vi "SortColumnEntriesIntoSections.vi"(1 "Array":refnum<class "ClickableText.lvclass">[](array[class])) -> (0 "Sorted Array":T1(array[cluster]))   [LabVIEW 2009, in "NavScreen.lvlib"]
uses:
  NavScreen.lvlib
  Classes/ClickableText/ClickableText.lvclass
  Classes/Link/Link.lvclass
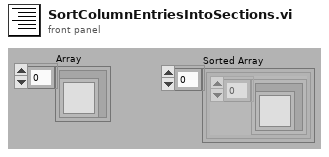
[diagram p1: front panel]
types:
  T1 = cluster{refnum<class "ClickableText.lvclass">[]}[]
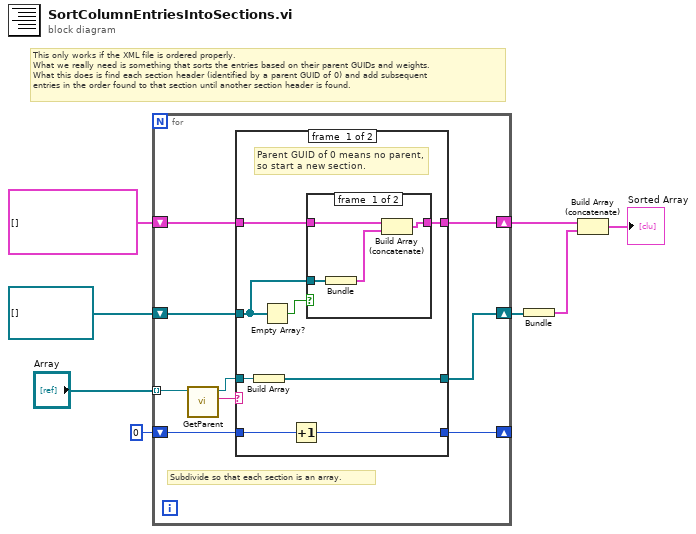
[diagram p0: block diagram]
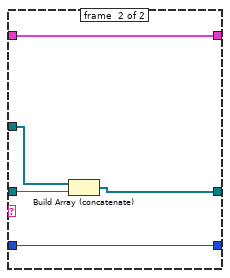
[diagram p3: hidden frame]
diagram:
  # "This only works if the XML file is ordered properly.\nWhat we really need is something that sorts the entries based on their parent GUIDs and weights.\nWhat this does is find each section header (identified by a parent GUID of 0) and add subsequent\nentries in the order found to that section until another section header is found."
  n1 = for {
    tunnel: "Array" -> [w10] mode=indexing
    shift-right: [w13] -> w6
    shift-left: refnum<class "ClickableText.lvclass">[] [] -> [w14]
    shift-right: [w15] -> _
    shift-left: 0 -> [w16]
    shift-right: [w12] -> w5
    shift-left: T1 [] -> [w11]
    # "Subdivide so that each section is an array."
    n2 = call "GetParent.vi"("Link in"=w10) -> ("parent GUID"=w17:string, "Link out"=w9:refnum<class "ClickableText.lvclass">)  [unwired: 8 in, 1 out]
    n3 = case shown="\"0\"" w17 {
      tunnel: w16 -> [w25 w32]
      tunnel: [w24 w32] -> w15
      tunnel: w14 -> [w21 w35]
      tunnel: w9 -> [w23 w34]
      tunnel: [w22 w33] -> w13
      tunnel: [w19 w31] -> w12
      tunnel: w11 -> [w18 w31]
      frame #0 {
        # "Parent GUID of 0 means no parent,\nso start a new section."
        n4 = Build Array(w23) -> (w22:refnum<class "ClickableText.lvclass">[])
        n5 = Empty Array?(array=w21) -> (empty?=w20:bool)
        n6 = Increment(x=w25) -> (x+1=w24:i32)
        n7 = case shown="False" w20 {
          tunnel: w21 -> [w29 _]
          tunnel: [w27 w30] -> w19
          tunnel: w18 -> [w26 w30]
          frame #0 {
            n8 = Bundle(w29) -> (w28:cluster{refnum<class "ClickableText.lvclass">[]})  [unwired: 1 in]
            n9 = Build Array (concatenate)(w26, w28) -> (w27:T1)
          }
          frame #1 {
          }
        }
      }
      frame #1 {
        n10 = Build Array (concatenate)(w35, w34) -> (w33:refnum<class "ClickableText.lvclass">[])
      }
    }
  }
  n11 = Bundle(w6) -> (w7:cluster{refnum<class "ClickableText.lvclass">[]})  [unwired: 1 in]
  n12 = Build Array (concatenate)(w5, w7) -> (→"Sorted Array":T1)
